vi "ReadValByRefEnumU16.vi"(0 "Control Ref":refnum<vi>, 2 "Type In":u16, 11 "error in":errorcluster caption="entrée d'erreur") -> (4 "Chaînes []":string[](array[string]), 6 "Valeur":u16, 8 "StringAtIdx":string, 15 "error out":errorcluster caption="sortie d'erreur")   [LabVIEW 2019]
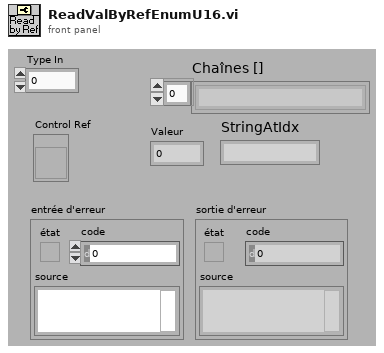
[diagram p1: front panel]
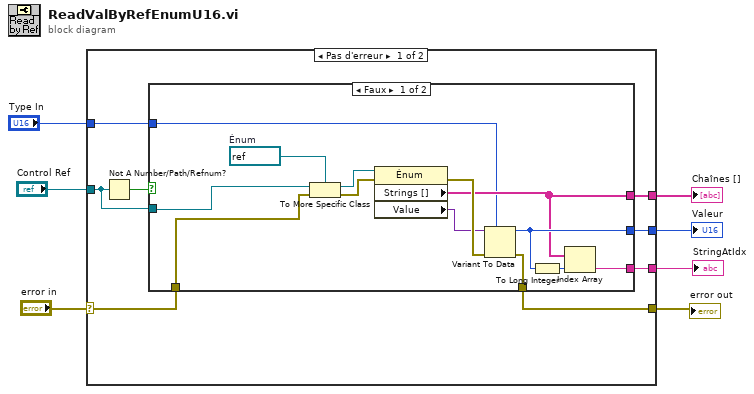
[diagram p0: block diagram]
diagram:
  n1 = case shown="Pas d'erreur" "error in" {
    selector: "error in" -> [w12 w30]
    tunnel: "Control Ref" -> [w14 _]
    tunnel: [w13 _] -> w6
    tunnel: [w11 w30] -> w4
    tunnel: [w10 _] -> w3
    tunnel: [w9 _] -> w2
    tunnel: "Type In" -> [w8 _]
    frame No Error {
      n2 = Not A Number/Path/Refnum?(number/path/refnum=w14) -> (NaN/Path/Refnum?=w15:bool)
      n3 = case shown="Faux" w15 {
        tunnel: w14 -> [w19 _]
        tunnel: [w26 _] -> w13
        tunnel: w12 -> [w18 w29]
        tunnel: [w28 w29] -> w11
        tunnel: [w23 _] -> w10
        tunnel: [w25 _] -> w9
        tunnel: w8 -> [w17 _]
        frame False {
          w20 = refnum<vi> refnum  # Énum
          n4 = To More Specific Class(target class=w20, reference=w19, error in=w18) -> (specific class reference=w22:refnum<vi>, error out=w21:errorcluster)
          n5 = property class="Énum"(reference=w22, error in=w21) -> (error out=w27:errorcluster, "Strings []"=w23:string[], "Value"=w16:variant)  [unwired: 1 out]
          n6 = Variant To Data(error in=w27, type=w17, Variant=w16) -> (data=w26:u16, error out=w28:errorcluster)
          n7 = To Long Integer(number=w26) -> (32bit integer=w24:i32)
          n8 = Index Array(array=w23, index=w24) -> (element=w25:string)
        }
        frame True {
        }
      }
    }
    frame Error {
    }
  }
  "Valeur" <- w6
  "error out" <- w4
  "Chaînes []" <- w3
  "StringAtIdx" <- w2
